vi "Close.vi"(8 "error in (no error)":errorcluster, 11 "Hart in":refnum<class "HART.lvclass">) -> (0 "error out":errorcluster, 3 "Hart out":refnum<class "HART.lvclass">)   [LabVIEW 2016, in "HART.lvclass"]
uses:
  HART.lvclass
  HART.lvclass/HART.ctl
  Protocol Class/Protocol.lvclass
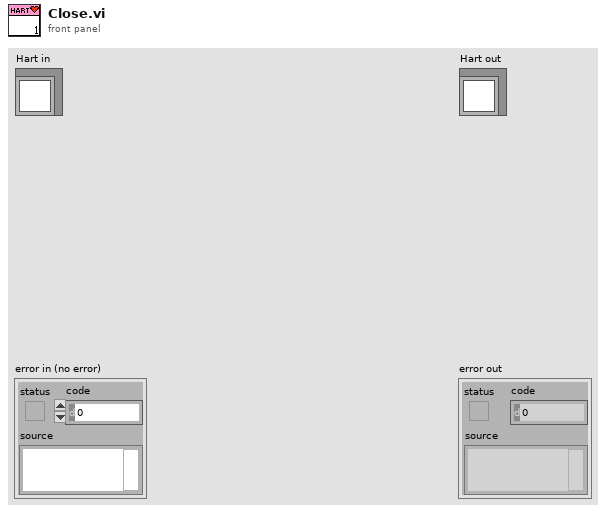
[diagram p1: front panel]
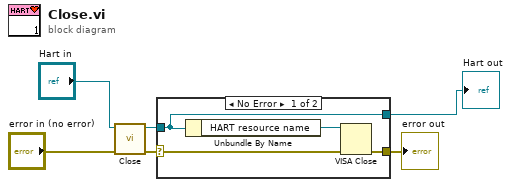
[diagram p0: block diagram]
diagram:
  n1 = call-parent "Close.vi"("error in (no error)"="error in (no error)", "Protocol in"="Hart in") -> ("error out"=w4:errorcluster, "Protocol out"=w2:refnum<class "HART.lvclass">)  [unwired: 8 in]
  n2 = case shown="No Error" w4 {
    selector: w4 -> [w9 w12]
    tunnel: [w8 w12] -> w3
    tunnel: w2 -> [w7 w11]
    tunnel: [w7 w11] -> w1
    frame No Error {
      n3 = Unbundle By Name(w7) -> ("HART resource name"=w10:refnum<visa-resource-name>)
      n4 = VISA Close(VISA resource name=w10, error in (no error)=w9) -> (error out=w8:errorcluster)
    }
    frame Error {
    }
  }
  "error out" <- w3
  "Hart out" <- w1
